vi "DistanceForm.vi"(8 "Center Y":dbl, 9 "Center X":dbl, 10 "Current Y":dbl, 11 "Current X":dbl) -> (3 "Distance":dbl)   [LabVIEW 2015]
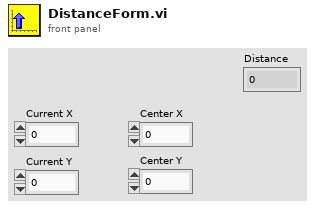
[diagram p1: front panel]
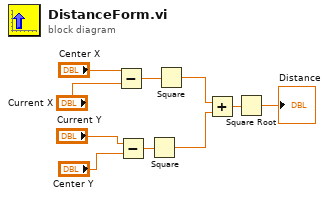
[diagram p0: block diagram]
diagram:
  n1 = Subtract(x="Center X", y="Current X") -> (x-y=w6:dbl)
  n2 = Subtract(x="Current Y", y="Center Y") -> (x-y=w5:dbl)
  n3 = Square(x=w5) -> (x^2=w3:dbl)
  n4 = Square(x=w6) -> (x^2=w4:dbl)
  n5 = Add(x=w4, y=w3) -> (x+y=w2:dbl)
  n6 = Square Root(x=w2) -> (sqrt(x)=→"Distance":dbl)
